vi "Calculate and Compare CRC.vi"(8 "Error In (No Error)":errorcluster, 11 "Sensor Response":string) -> (0 "Error Out":errorcluster, 1 "CRC Correct?":bool, 2 "Calculated CRC":string, 3 "Sent CRC":string)   [LabVIEW 2016, in "SDI-12.lvlib"]
doc: "Calculates the CRC using the algorithm for SDI-12 version 1.3. The algorithm used to calculate it can be found at http://www.sdi-12.org/. For your convenience, the CRC algorithm is commented in C style above the equivalent LabVIEW code."
uses:
  SDI-12.lvlib
panel:
  in  "CRC":u16 format="%x"
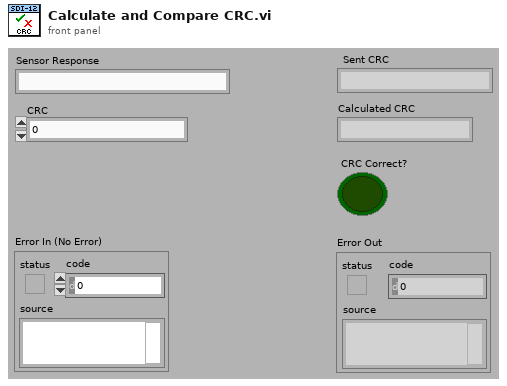
[diagram p1: front panel]
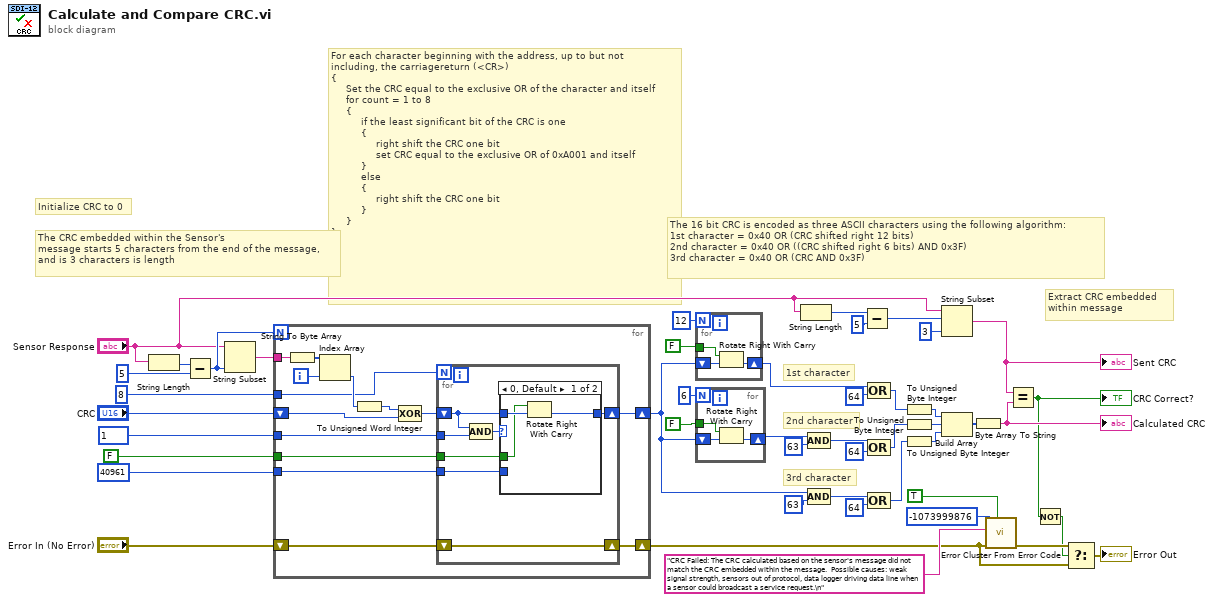
[diagram p0: block diagram]
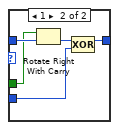
[diagram p2: hidden frame]
diagram:
  # "Extract CRC embedded \nwithin message"
  # "3rd character"
  # "2nd character"
  # "1st character"
  # "The 16 bit CRC is encoded as three ASCII characters using the following algorithm:\n1st character = 0x40 OR (CRC shifted right 12 bits)\n2nd character = 0x40 OR ((CRC shifted right 6 bits) AND 0x3F)\n3rd character = 0x40 OR (CRC AND 0x3F)"
  # "For each character beginning with the address, up to but not \nincluding, the carriagereturn (<CR>)\n{\n     Set the CRC equal to the exclusive OR of the character and itself\n     for count = 1 to 8\n     {\n          if the least significant bit of the CRC is one\n          {\n               right shift the CRC one bit\n               set CRC equal to the exclusive OR of 0xA001 and itself\n          }\n          else\n          {\n               right shift the CRC one bit\n          }\n     }\n}"
  # "Initialize CRC to 0"
  # "The CRC embedded within the Sensor's\nmessage starts 5 characters from the end of the message,\nand is 3 characters is length"
  n1 = String Length(string="Sensor Response") -> (length=w42:i32)
  n2 = Subtract(x=w42, y=5) -> (x-y=w45:i32)
  n3 = String Subset(string="Sensor Response", length (rest)=w45) -> (substring=w44:string)  [unwired: 1 in]
  n4 = for {
    N: w45 -> [_]
    shift-right: [w57] -> w7
    shift-left: "Error In (No Error)" -> [w58]
    tunnel: w44 -> [w56]
    shift-right: [w51] -> w13
    shift-left: "CRC" -> [w53]
    tunnel: u16 1 ("CRC") -> [w50]
    tunnel: u16 40961 ("value") -> [w49]
    tunnel: FALSE ("carry") -> [w48]
    tunnel: 8 -> [w47]
    i -> [w55]
    n5 = String To Byte Array(string=w56) -> (unsigned byte array=w60:u8[])
    n6 = Index Array(array=w60, index=w55) -> (element=w54:u8)
    n7 = To Unsigned Word Integer(number=w54) -> (unsigned 16bit integer=w59:u16)
    n8 = Compound Arithmetic op=XOR(w59, w53) -> (w52:u16)
    n9 = for {
      N: w47 -> [_]
      shift-right: [w66] -> w57
      shift-left: w58 -> [w66]
      shift-right: [w65] -> w51
      shift-left: w52 -> [w64]
      tunnel: w50 -> [w63]
      tunnel: w49 -> [w62]
      tunnel: w48 -> [w61]
      n10 = Compound Arithmetic op=AND(w64, w63) -> (w67:u16)
      n11 = case shown="0, Default" w67 {
        tunnel: w64 -> [w70 w75]
        tunnel: [w69 w73] -> w65
        tunnel: w62 -> [_ w72]
        tunnel: w61 -> [w68 w71]
        frame 0, Default {
          n12 = Rotate Right With Carry(2:w70, 3:w68) -> (0:w69:u16)  [unwired: 1 out]
        }
        frame 1 {
          n13 = Rotate Right With Carry(2:w75, 3:w71) -> (0:w74:u16)  [unwired: 1 out]
          n14 = Compound Arithmetic op=XOR(w74, w72) -> (w73:u16)
        }
      }
    }
  }
  n15 = for {
    N: 12 -> [_]
    tunnel: FALSE ("carry") -> [w78]
    shift-right: [w76] -> w33
    shift-left: w13 -> [w77]
    n16 = Rotate Right With Carry(2:w77, 3:w78) -> (0:w76:u16)  [unwired: 1 out]
  }
  n17 = for {
    N: 6 -> [_]
    tunnel: FALSE ("carry") -> [w81]
    shift-right: [w79] -> w25
    shift-left: w13 -> [w80]
    n18 = Rotate Right With Carry(2:w80, 3:w81) -> (0:w79:u16)  [unwired: 1 out]
  }
  n19 = String Length(string="Sensor Response") -> (length=w15:i32)
  n20 = Compound Arithmetic op=AND(w25, u16 63 ("value")) -> (w24:u16)
  n21 = Compound Arithmetic op=AND(w13, u16 63 ("value")) -> (w22:u16)
  n22 = Subtract(x=w15, y=5) -> (x-y=w18:i32)
  n23 = Compound Arithmetic op=OR(w33, u16 64 ("value")) -> (w19:u16)
  n24 = Compound Arithmetic op=OR(w24, u16 64 ("value")) -> (w30:u16)
  n25 = Compound Arithmetic op=OR(w22, u16 64 ("value")) -> (w3:u16)
  n26 = To Unsigned Byte Integer(number=w19) -> (unsigned 8bit integer=w32:u8)
  n27 = To Unsigned Byte Integer(number=w30) -> (unsigned 8bit integer=w21:u8)
  n28 = To Unsigned Byte Integer(number=w3) -> (unsigned 8bit integer=w20:u8)
  n29 = String Subset(string="Sensor Response", offset (0)=w18, length (rest)=3 ("length (rest)")) -> (substring=w5:string)
  "Sent CRC" <- w5
  n30 = Build Array(w32, w21, w20) -> (w31:u8[])
  n31 = Byte Array To String(unsigned byte array=w31) -> (string=w4:string)
  "Calculated CRC" <- w4
  n32 = call <vilib>:"Error Cluster From Error Code.vi"("show call chain? (False)"=TRUE ("Error?"), "error in (no error)"=w7, "error message (\"\")"="CRC Failed: The CRC calculated based on the sensor's message did not match the CRC embedded within the message.  Possible causes: weak signal strength, sensors out of protocol, data logger driving data line when a sensor could broadcast a service request.\n" ("error message (\"\")"), "error code (0)"=-1073999876 ("error code")) -> ("error out"=w9:errorcluster)  [unwired: 5 in]
  n33 = Equal?(x=w5, y=w4) -> (x = y?=w2:bool)
  "CRC Correct?" <- w2
  n34 = Not(x=w2) -> (.not. x?=w1:bool)
  n35 = Select(t=w9, s=w1, f=w7) -> (s? t:f=→"Error Out":errorcluster)
